vi "AutoMeasurement.vi"(6 "index":i32, 9 "CTRL HWSync":refnum<notifier>, 10 "HAL":refnum<queue>, 11 "Queue in":refnum<queue>) -> ()   [LabVIEW 2014]
uses:
  APIs/Data Queue/Control Data Cluster.ctl
  APIs/Message Queue/Message Cluster.ctl
  APIs/Message Queue/Enqueue Message (Single).vi
  APIs/Message Queue/Enqueue Message (Array).vi
  APIs/Data Queue/WINFAS 2 Data Queue.lvlib
  APIs/Message Queue/WINFAS 2 Message Queue.lvlib
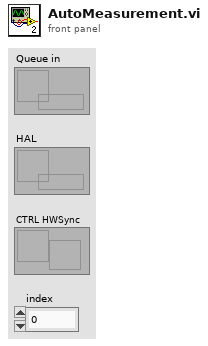
[diagram p1: front panel]
types:
  T1 = typedef "WINFAS 2 Data Queue.lvlib/Control Data Cluster.ctl" = cluster{"Encoder":sgl, "DI":bool[], "DO":bool[]}
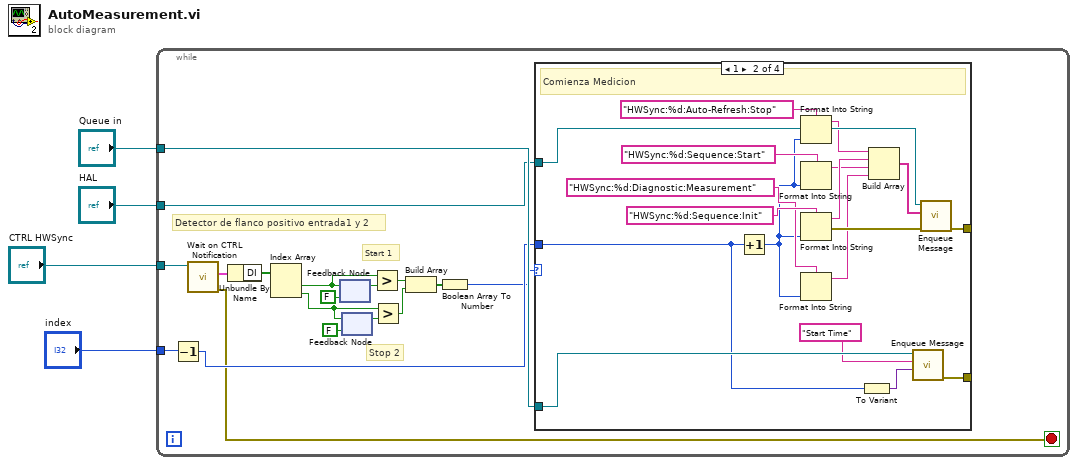
[diagram p0: block diagram]
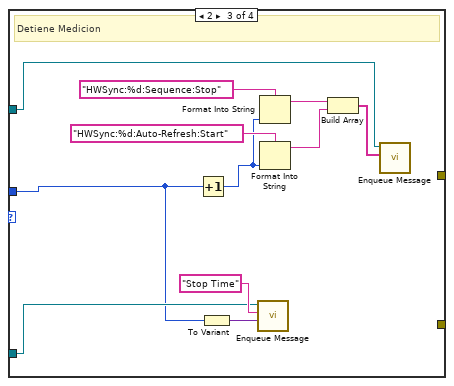
[diagram p3: hidden frame]
diagram:
  n1 = while {
    tunnel: "Queue in" -> [w10]
    tunnel: "HAL" -> [w9]
    tunnel: "CTRL HWSync" -> [w17]
    tunnel: "index" -> [w8]
    stop <- w5 stop-if-true
    # "Detector de flanco positivo entrada1 y 2"
    # "Stop 2"
    # "Start 1"
    n2 = Decrement(x=w8) -> (x-1=w7:i32)
    n3 = call "Wait on CTRL Notification.vi"("CTRL Data Notifier in"=w17) -> ("error out"=w5:errorcluster, "Control Data"=w22:T1)  [unwired: 7 in, 2 out]
    n4 = Unbundle By Name(w22) -> ("DI"=w21:bool[])
    n5 = Index Array(array=w21) -> (element #1=w19:bool, element #2=w14:bool)  [unwired: 2 in]
    n6 = feedback-in #1(w19) -> ()
    n7 = feedback #1(FALSE ("Boolean")) -> (w18:bool)
    n8 = feedback #2(FALSE ("Boolean")) -> (w16:bool)
    n9 = feedback-in #2(w14) -> ()
    n10 = Greater?(x=w19, y=w18) -> (0:w13:bool)
    n11 = Greater?(x=w14, y=w16) -> (0:w12:bool)
    n12 = Build Array(w13, w12) -> (w11:bool[])
    n13 = Boolean Array To Number(Boolean array=w11) -> (number=w6:u32)
    n14 = case shown="1" w6 {
      tunnel: [_ w39 _ _] -> _
      tunnel: w9 -> [_ w38 w43 _]
      tunnel: w7 -> [_ w24 w41 _]
      tunnel: w10 -> [_ w28 w42 _]
      tunnel: [_ w25 _ _] -> _
      frame 0, Default {
      }
      frame 1 {
        # "Comienza Medicion"
        n15 = Increment(x=w24) -> (x+1=w29:i32)
        n16 = Format Into String(format string="HWSync:%d:Auto-Refresh:Stop", w29) -> (resulting string=w23:string)  [unwired: 2 in, 1 out]
        n17 = Format Into String(format string="HWSync:%d:Sequence:Start", w29) -> (resulting string=w30:string)  [unwired: 2 in, 1 out]
        n18 = Format Into String(format string="HWSync:%d:Sequence:Init", w29) -> (resulting string=w33:string, error out=w37:errorcluster)  [unwired: 2 in]
        n19 = Format Into String(format string="HWSync:%d:Diagnostic:Measurement", w29) -> (resulting string=w32:string)  [unwired: 2 in, 1 out]
        n20 = To Variant(anything=w24) -> (Variant=w26:variant)
        n21 = Build Array(w23, w33, w30, w32) -> (w36:string[])
        n22 = call-poly "Enqueue Message.vi"("Message Data"=w26, "Message"="Start Time", "Message Queue"=w28) -> ("error out"=w25:errorcluster)  [unwired: 7 in, 1 out]
        n23 = call-poly "Enqueue Message.vi"("error in (no error)"=w37, "Message Array"=w36, "Message Queue"=w38) -> ("error out"=w39:errorcluster)  [unwired: 7 in, 1 out]
      }
      frame 2 {
        # "Detiene Medicion"
        n24 = Increment(x=w41) -> (x+1=w47:i32)
        n25 = To Variant(anything=w41) -> (Variant=w46:variant)
        n26 = call-poly "Enqueue Message.vi"("Message Data"=w46, "Message"="Stop Time", "Message Queue"=w42) -> ()  [unwired: 7 in, 2 out]
        n27 = Format Into String(format string="HWSync:%d:Sequence:Stop", w47) -> (resulting string=w45:string)  [unwired: 2 in, 1 out]
        n28 = Format Into String(format string="HWSync:%d:Auto-Refresh:Start", w47) -> (resulting string=w48:string)  [unwired: 2 in, 1 out]
        n29 = Build Array(w45, w48) -> (w51:string[])
        n30 = call-poly "Enqueue Message.vi"("Message Array"=w51, "Message Queue"=w43) -> ()  [unwired: 8 in, 2 out]
      }
      frame 3 {
      }
    }
  }
